vi "Water Tunnel Front Panel.vi"() -> ()   [LabVIEW 2019, in "Results.lvlib" / "Water Tunnel Results.lvclass"]
uses:
  Water Tunnel Results.lvclass
  Water Tunnel Results.lvclass/Water Tunnel Results.ctl
  Test Stands/Water Tunnel/Water Tunnel Test Stand.lvclass
panel:
  out "Traverse Message":string
  out "Traverse Raw String":string
  out "Wing Aligned?":bool=TRUE caption="Wing"
  out "Probe Aligned?":bool=TRUE caption="Probe"
  in  "Trav SetP":T1
  in  "Trav Probe Set?":bool caption="Probe Traverse"
  in  "Trav Wing Set?":bool caption="Wing Traverse"
  in  "Pump Load":dbl caption="Pump Load, %" step=10.0 format="%#.2f"
  out "p8":dbl format="%#.2f"
  out "p7":dbl format="%#.2f"
  out "p6":dbl format="%#.2f"
  out "p4":dbl format="%#.2f"
  out "p2":dbl format="%#.2f"
  out "p1":dbl format="%#.2f"
  out "p3":dbl format="%#.2f"
  out "p5":dbl format="%#.2f"
  out "Angle U":dbl format="%#.4f"
  out "Angle":dbl caption="Pitch" format="%#.2f"
  out "Data":waveform(dbl)[](graph) caption="Pressures"
  # "V"
  # "deg"
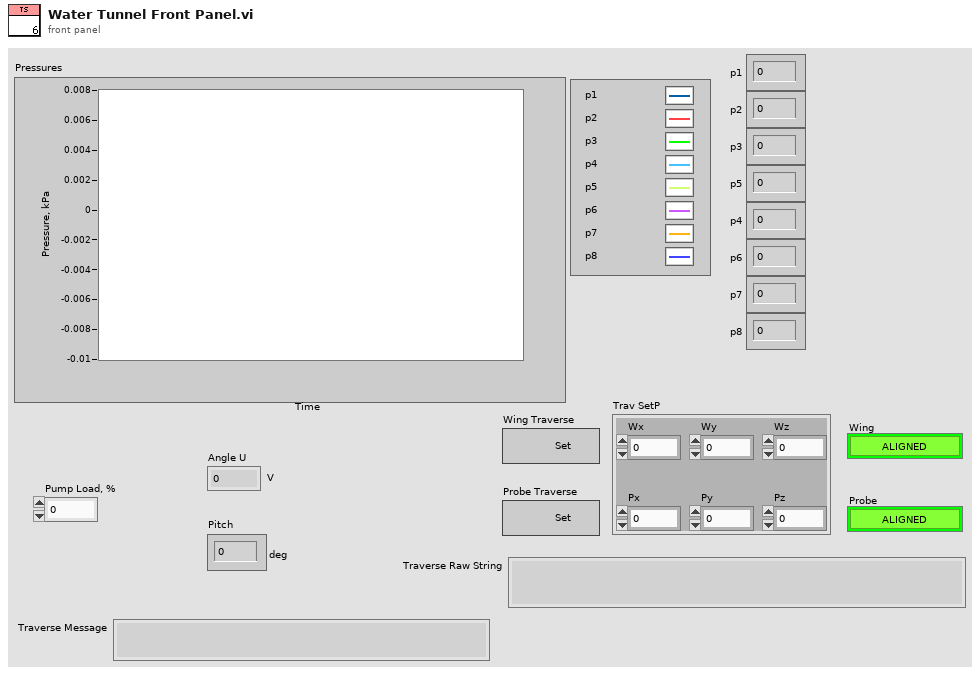
[diagram p1: front panel]
types:
  T1 = cluster{"Wx":dbl, "Wy":dbl, "Wz":dbl, "Px":dbl, "Py":dbl, "Pz":dbl}
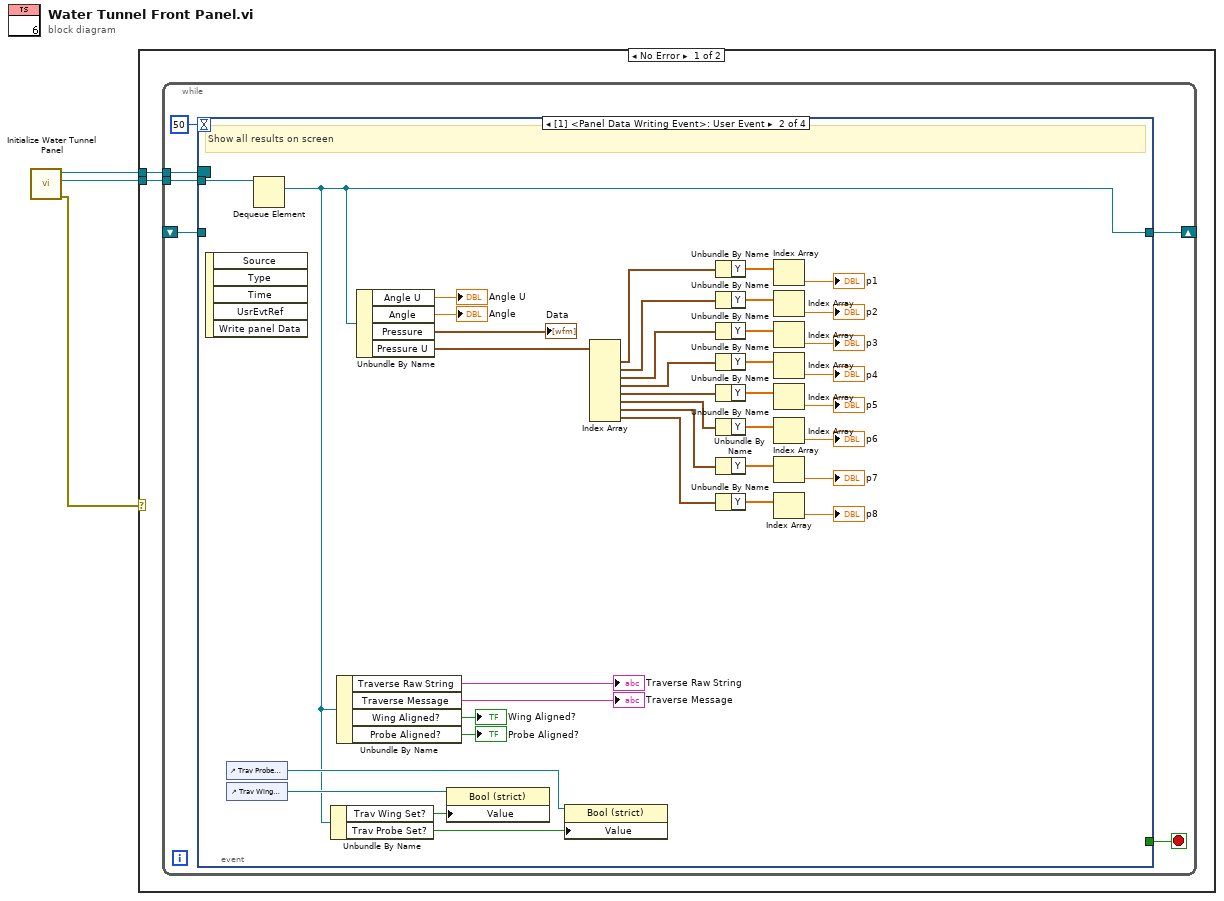
[diagram p0: block diagram]
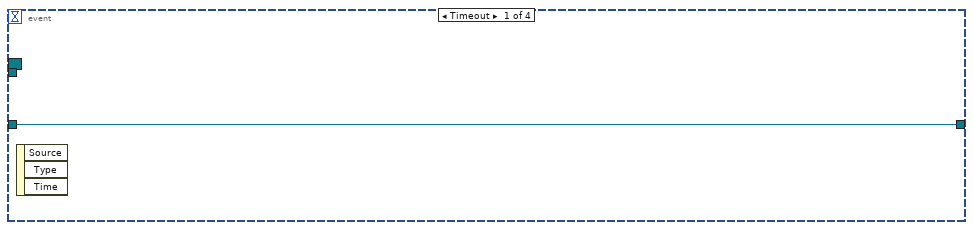
[diagram p2: hidden frame]
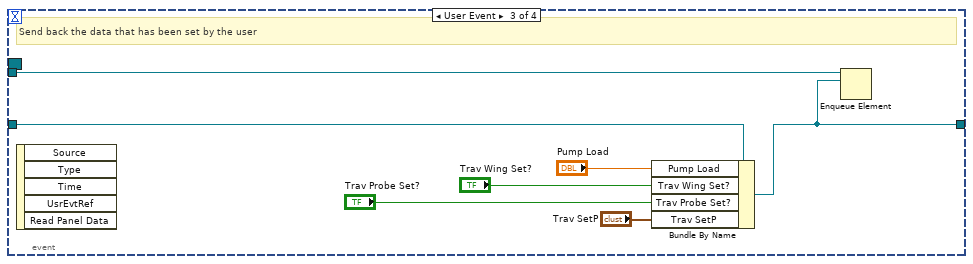
[diagram p3: hidden frame]
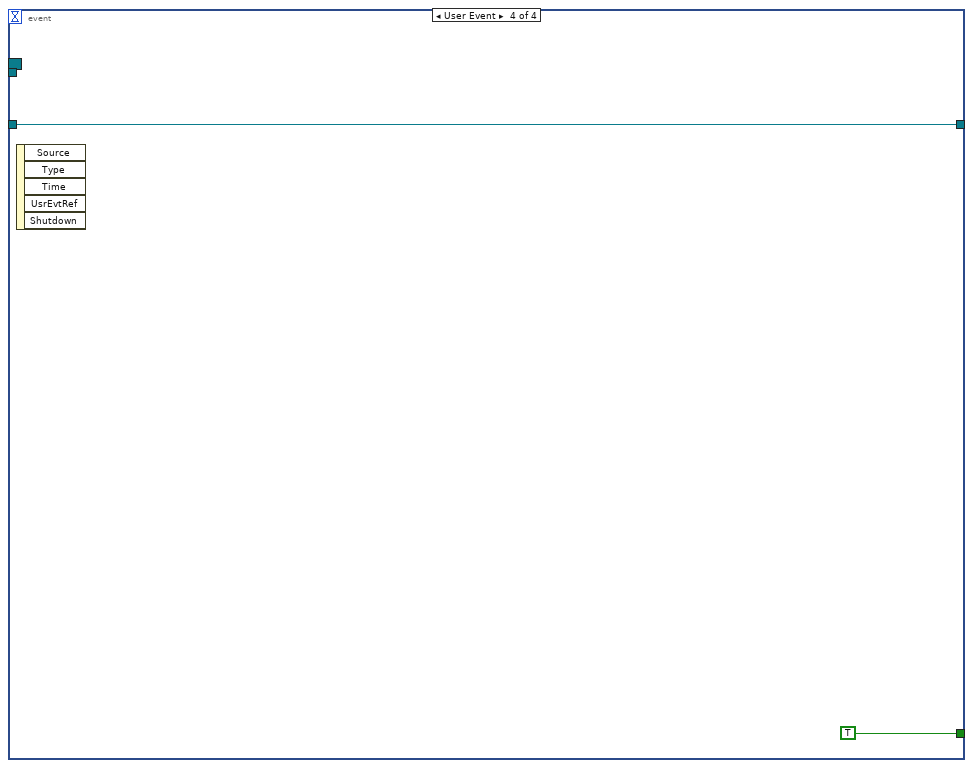
[diagram p4: hidden frame]
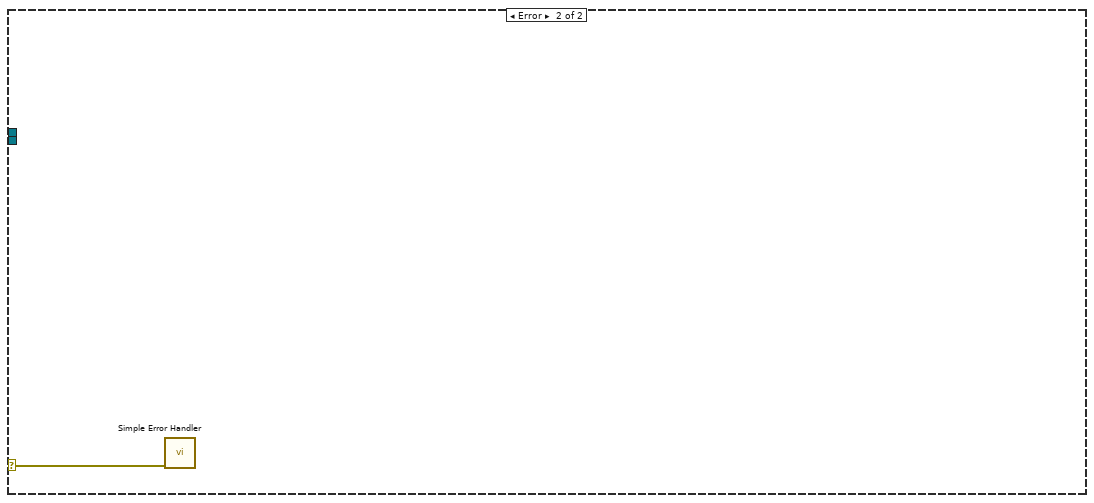
[diagram p5: hidden frame]
diagram:
  n1 = call "Initialize Water Tunnel Panel.vi"() -> ("error out"=w1:errorcluster, "Water Tunnel Results queue out"=w2:refnum<queue>, "Event Registration Refnum"=w3:refnum<event-registration>)  [unwired: 9 in]
  n2 = case shown="No Error" w1 {
    selector: w1 -> [_ w60]
    tunnel: w3 -> [w5 _]
    tunnel: w2 -> [w4 _]
    frame No Error {
      n3 = while {
        tunnel: w5 -> [w10]
        tunnel: w4 -> [w9]
        shift-right: [w7] -> _
        shift-left: _ -> [w6]
        stop <- w11 stop-if-true
        n4 = event shown="[1] <Panel Data Writing Event>: User Event" {
          selector: w10 -> [_ _ _ _]
          dyn-events: _ -> [_ _ _ _]
          timeout: 50 -> [_ _ _ _]
          tunnel: [_ _ _ TRUE] -> w11
          tunnel: w9 -> [_ w50 w57 _]
          tunnel: [w12 w19 w55 w58] -> w7
          tunnel: w6 -> [w12 _ w56 w58]
          event Timeout {
            n5 = event-data() -> ()  [unwired: 1 in, 3 out]
          }
          event User Event {
            # "Show all results on screen"
            n6 = event-data() -> ()  [unwired: 1 in, 5 out]
            n7 = control-ref of="Trav Probe Set?"() -> (w22:refnum<vi>)
            n8 = control-ref of="Trav Wing Set?"() -> (w23:refnum<vi>)
            n9 = Dequeue Element(queue=w50) -> (element=w19:refnum<class "Water Tunnel Results.lvclass">)  [unwired: 2 in, 3 out]
            n10 = Unbundle By Name(w19) -> ("Trav Wing Set?"=w21:bool, "Trav Probe Set?"=w20:bool)
            n11 = Unbundle By Name(w19) -> ("Traverse Raw String"=→"Traverse Raw String":string, "Traverse Message"=→"Traverse Message":string, "Wing Aligned?"=→"Wing Aligned?":bool, "Probe Aligned?"=→"Probe Aligned?":bool)
            n12 = Unbundle By Name(w19) -> ("Angle U"=→"Angle U":dbl, "Angle"=→"Angle":dbl, "Pressure"=→"Data":waveform(dbl)[], "Pressure U"=w25:waveform(dbl)[])
            n13 = property class="Bool (strict)"(reference=w23, "Value"=w21) -> ()  [unwired: 1 in, 2 out]
            n14 = property class="Bool (strict)"(reference=w22, "Value"=w20) -> ()  [unwired: 1 in, 2 out]
            n15 = Index Array(array=w25) -> (element #1=w49:waveform(dbl), element #2=w46:waveform(dbl), element #3=w43:waveform(dbl), element #4=w41:waveform(dbl), element #5=w39:waveform(dbl), element #6=w28:waveform(dbl), element #7=w27:waveform(dbl), element #8=w26:waveform(dbl))  [unwired: 8 in]
            n16 = Unbundle By Name(w49) -> ("Y"=w48:dbl[])
            n17 = Unbundle By Name(w46) -> ("Y"=w45:dbl[])
            n18 = Unbundle By Name(w43) -> ("Y"=w42:dbl[])
            n19 = Unbundle By Name(w41) -> ("Y"=w40:dbl[])
            n20 = Unbundle By Name(w39) -> ("Y"=w38:dbl[])
            n21 = Unbundle By Name(w28) -> ("Y"=w33:dbl[])
            n22 = Unbundle By Name(w27) -> ("Y"=w32:dbl[])
            n23 = Unbundle By Name(w26) -> ("Y"=w29:dbl[])
            n24 = Index Array(array=w48) -> (element=→"p1":dbl)  [unwired: 1 in]
            n25 = Index Array(array=w45) -> (element=→"p2":dbl)  [unwired: 1 in]
            n26 = Index Array(array=w42) -> (element=→"p3":dbl)  [unwired: 1 in]
            n27 = Index Array(array=w40) -> (element=→"p4":dbl)  [unwired: 1 in]
            n28 = Index Array(array=w38) -> (element=→"p5":dbl)  [unwired: 1 in]
            n29 = Index Array(array=w33) -> (element=→"p6":dbl)  [unwired: 1 in]
            n30 = Index Array(array=w32) -> (element=→"p7":dbl)  [unwired: 1 in]
            n31 = Index Array(array=w29) -> (element=→"p8":dbl)  [unwired: 1 in]
          }
          event User Event {
            # "Send back the data that has been set by the user"
            n32 = event-data() -> ()  [unwired: 1 in, 5 out]
            n33 = Bundle By Name(cluster=w56, "Pump Load"="Pump Load", "Trav Wing Set?"="Trav Wing Set?", "Trav Probe Set?"="Trav Probe Set?", "Trav SetP"="Trav SetP") -> (w55:refnum<class "Water Tunnel Results.lvclass">)
            n34 = Enqueue Element(queue=w57, element=w55) -> ()  [unwired: 2 in, 3 out]
          }
          event User Event {
            n35 = event-data() -> ()  [unwired: 1 in, 5 out]
          }
        }
      }
    }
    frame Error {
      n36 = call <vilib>:"Simple Error Handler.vi"("error in (no error)"=w60) -> ()  [unwired: 4 in, 5 out]
    }
  }
